vi "Do Get Cond Terminal.vi"(8 "error in (no error)":errorcluster, 10 "get_loop_conditional_terminal Argument":T3, 11 "Data Cluster in":T1) -> (0 "error out":errorcluster, 2 "get_loop_conditional_terminal (Reply Payload)":T2, 3 "Data Cluster out":T1)   [LabVIEW 2025, in "Scripting Server.lvlib"]
uses:
  Scripting Server.lvlib
  Module Data--cluster.ctl
  get_loop_conditional_terminal Argument--cluster.ctl
  get_loop_conditional_terminal (Reply Payload)--cluster.ctl
  <vilib>/Utility/error.llb/Error Cluster From Error Code.vi
  <vilib>/ErrorRing/Error Ring.xnode
panel:
  out "Class Name":string
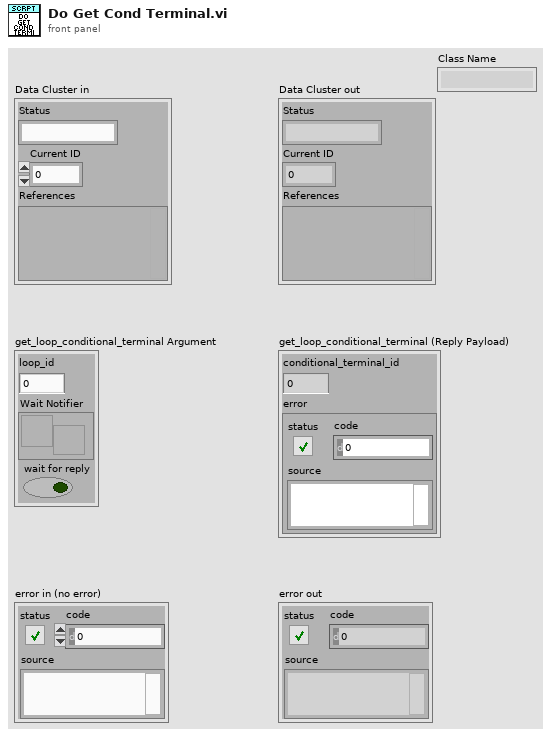
[diagram p1: front panel]
types:
  T1 = typedef "Scripting Server.lvlib/Module Data--cluster.ctl" = cluster{"Status":string, "Current ID":i32, "References":variant}
  T2 = typedef "Scripting Server.lvlib/get_loop_conditional_terminal (Reply Payload)--cluster.ctl" = cluster{"conditional_terminal_id":i32, "error":errorcluster}
  T3 = typedef "Scripting Server.lvlib/get_loop_conditional_terminal Argument--cluster.ctl" = cluster{"loop_id":i32, "Wait Notifier":refnum<notifier>, "wait for reply":bool}
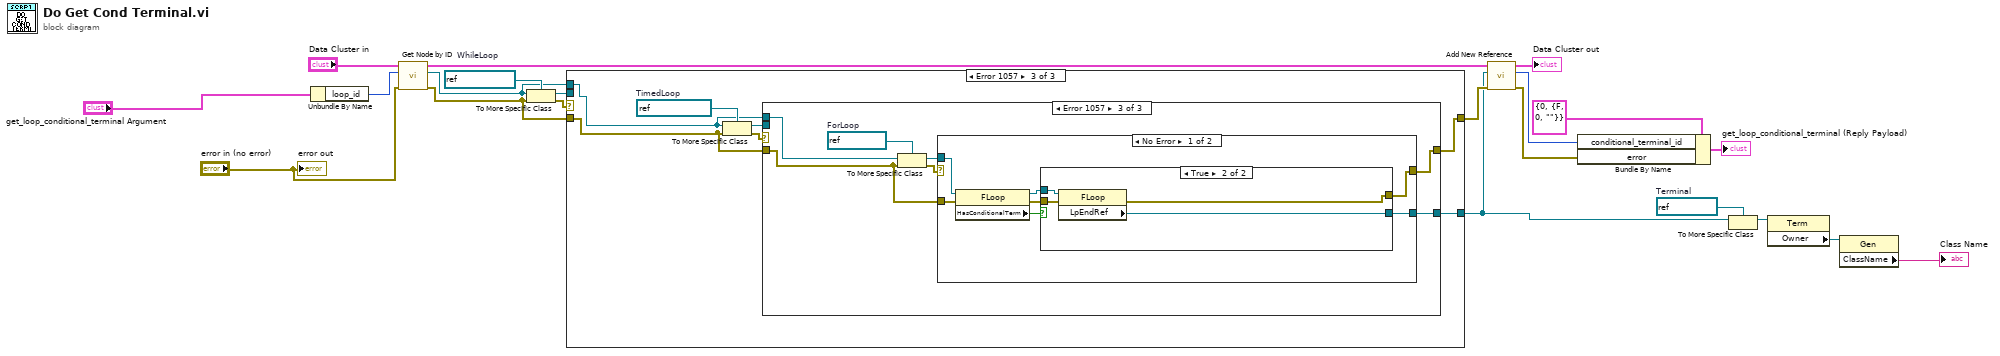
[diagram p0: block diagram]
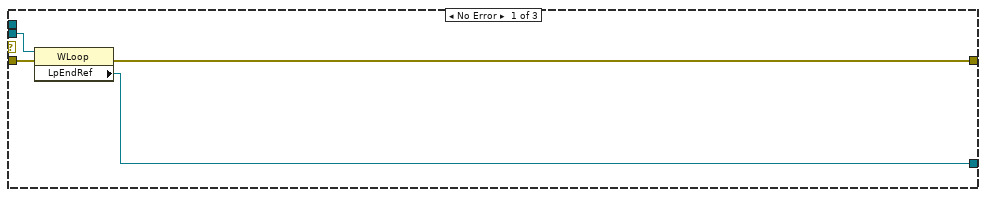
[diagram p2: hidden frame]
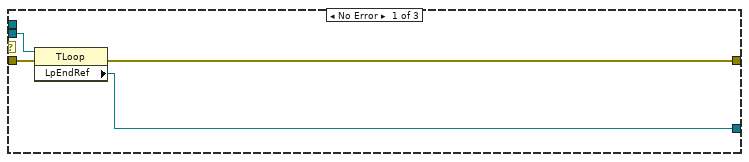
[diagram p4: hidden frame]
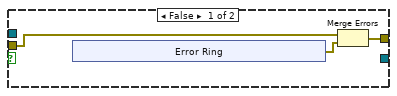
[diagram p6: hidden frame]
diagram:
  w3 = refnum<vi> refnum  # Terminal
  w16 = refnum<vi> refnum  # WhileLoop
  n1 = Unbundle By Name("get_loop_conditional_terminal Argument") -> ("loop_id"=w17:i32)
  n2 = call "Get Node by ID.vi"("error in (no error)"="error in (no error)", "ID"=w17, "Data Cluster in"="Data Cluster in") -> ("error out"=w6:errorcluster, "specific class reference"=w1:refnum<vi>, "Data Cluster out"=w11:T1)  [unwired: 6 in]
  n3 = To More Specific Class(target class=w16, reference=w1, error in=w6) -> (specific class reference=w15:refnum<vi>, error out=w7:errorcluster)
  n4 = case shown="Error 1057" w7 {
    tunnel: w15 -> [w25 _ _]
    tunnel: [w24 w26 w32] -> w14
    tunnel: [w23 _ w30] -> w8
    tunnel: w6 -> [w22 w26 w28]
    tunnel: w1 -> [_ _ w27]
    frame No Error {
      n5 = property class="WLoop"(reference=w25, error in=w22) -> (error out=w24:errorcluster, "LpEndRef"=w23:refnum<vi>)  [unwired: 1 out]
    }
    frame Default {
    }
    frame Error {
      w33 = refnum<vi> refnum  # TimedLoop
      n6 = To More Specific Class(target class=w33, reference=w27, error in=w28) -> (specific class reference=w31:refnum<vi>, error out=w29:errorcluster)
      n7 = case shown="Error 1057" w29 {
        tunnel: w28 -> [w37 w38 w41]
        tunnel: [w36 w38 w43] -> w32
        tunnel: w31 -> [w35 _ _]
        tunnel: [w34 _ w42] -> w30
        tunnel: w27 -> [_ _ w39]
        frame No Error {
          n8 = property class="TLoop"(reference=w35, error in=w37) -> (error out=w36:errorcluster, "LpEndRef"=w34:refnum<vi>)  [unwired: 1 out]
        }
        frame Default {
        }
        frame Error {
          w44 = refnum<vi> refnum  # ForLoop
          n9 = To More Specific Class(target class=w44, reference=w39, error in=w41) -> (specific class reference=w45:refnum<vi>, error out=w40:errorcluster)
          n10 = case shown="No Error" w40 {
            selector: w40 -> [_ w65]
            tunnel: w41 -> [w52 _]
            tunnel: w45 -> [w50 _]
            tunnel: [w49 w65] -> w43
            tunnel: [w46 _] -> w42
            frame No Error {
              n11 = property class="FLoop"(reference=w50, error in=w52) -> (reference out=w47:refnum<vi>, error out=w51:errorcluster, "HasConditionalTerm"=w48:bool)
              n12 = case shown="True" w48 {
                tunnel: w51 -> [w55 w64]
                tunnel: [w54 w63] -> w49
                tunnel: w47 -> [_ w62]
                tunnel: [_ w61] -> w46
                frame False {
                  n13 = xnode "Error Ring"() -> ("error out"=w53:errorcluster)
                  n14 = Merge Errors(w55, w53) -> (w54:errorcluster)
                }
                frame True {
                  n15 = property class="FLoop"(reference=w62, error in=w64) -> (error out=w63:errorcluster, "LpEndRef"=w61:refnum<vi>)  [unwired: 1 out]
                }
              }
            }
            frame Error {
            }
          }
        }
      }
    }
  }
  n16 = call "Add New Reference.vi"("error in (no error)"=w14, "Variant"=w8, "Data Cluster in"=w11) -> ("error out"=w12:errorcluster, "new reference"=w9:i32, "Data Cluster out 2"=→"Data Cluster out":T1)  [unwired: 6 in]
  n17 = Bundle By Name(cluster=T2 {"conditional_terminal_id"=0, "error"={"status"=FALSE, "code"=0, "source"=""}} ("get_loop_conditional_terminal (Reply Payload)"), "conditional_terminal_id"=w9, "error"=w12) -> (→"get_loop_conditional_terminal (Reply Payload)":T2)
  n18 = To More Specific Class(target class=w3, reference=w8) -> (specific class reference=w4:refnum<vi>)  [unwired: 1 in, 1 out]
  n19 = property class="Term"(reference=w4) -> ("Owner"=w5:refnum<vi>)  [unwired: 1 in, 2 out]
  n20 = property class="Gen"(reference=w5) -> ("ClassName"=→"Class Name":string)  [unwired: 1 in, 2 out]
  "error out" <- "error in (no error)"
